vi "get_level.vi"(8 "error in (no error)":errorcluster, 11 "Queue Log Provider in":refnum<class "Queue Log Provider.lvclass">) -> (0 "error out":errorcluster, 1 "level":T1 items=["OFF"=0, "FATAL"=100, "ERROR"=200, "WARN"=300, "INFO"=400, "DEBUG"=500, "TRACE"=600, "ALL"=65535], 3 "Queue Log Provider out":refnum<class "Queue Log Provider.lvclass">)   [LabVIEW 2019, in "LVCOOOP.lvlib" / "Support API.lvlib" / "Queue Log Provider.lvclass"]
uses:
  Queue Log Provider.lvclass
  Log Service/public/level.ctl
  Log Service/Log Service.lvclass
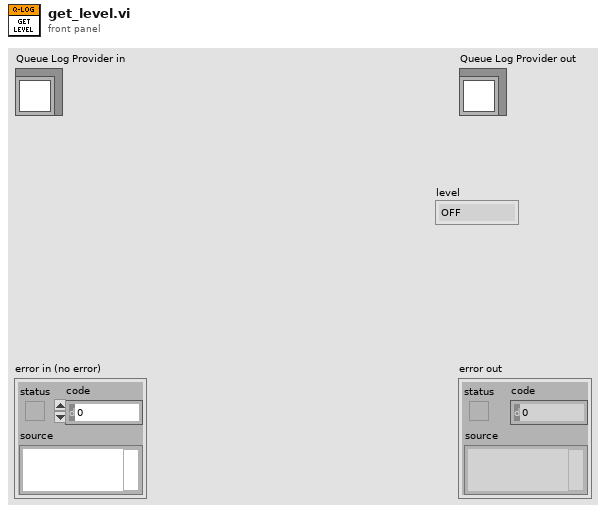
[diagram p1: front panel]
types:
  T1 = typedef "LVCOOOP.lvlib/Support API.lvlib/Log Service.lvclass/level.ctl" = u16
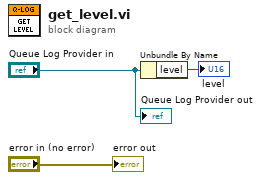
[diagram p0: block diagram]
diagram:
  n1 = Unbundle By Name("Queue Log Provider in") -> ("level"=→"level":T1)
  "error out" <- "error in (no error)"
  "Queue Log Provider out" <- "Queue Log Provider in"
